vi "Set Averaging.vi"(0 "VISA resource name":refnum<visa-resource-name>, 1 "IF bandwidth (5 : 3000 HZ)":u16(ring)=5 items=["10 HZ", "30 HZ", "100 HZ", "300 HZ", "1000 HZ", "3000 HZ"], 2 "smoothing (F : off)":bool, 5 "average (F : off)":bool, 9 "average factor (16)":u16=16 min=1 max=999, 11 "error in (no error)":errorcluster, 13 "smoothing aperature (1%)":sgl=1.0 min=0.05 max=20 format="%.2f") -> (4 "VISA resource name out":refnum<visa-resource-name>, 15 "error out":errorcluster)   [LabVIEW 2018, in "Agilent 87XX Series.lvlib"]
doc: "This Vi for the HP8753B Network Analyzer is used to set averaging, smoothing, and the IF bandwidth."
uses:
  Agilent 87XX Series.lvlib
panel:
  # "ON\nOFF"
  # "ON\nOFF"
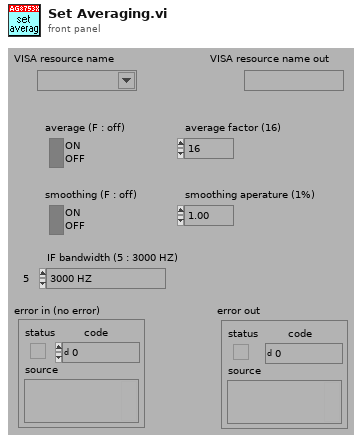
[diagram p1: front panel]
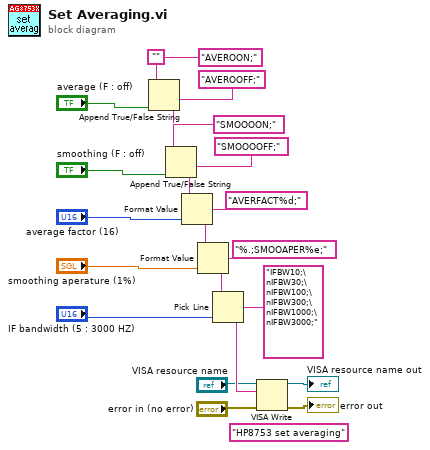
[diagram p0: block diagram]
diagram:
  (unwired) "HP8753 set averaging"
  n1 = Append True/False String(1:"average (F : off)", 2:"AVEROOFF;", 3:"AVEROON;", 4:"") -> (0:w16:string)
  n2 = Append True/False String(1:"smoothing (F : off)", 2:"SMOOOOFF;", 3:"SMOOOON;", 4:w16) -> (0:w14:string)
  n3 = Format Value(string ("")=w14, format string="AVERFACT%d;", value (0)="average factor (16)") -> (output string=w10:string)
  n4 = Format Value(string ("")=w10, format string="%.;SMOOAPER%e;", value (0)="smoothing aperature (1%)") -> (output string=w8:string)
  n5 = Pick Line(string ("")=w8, multi-line string="IFBW10;\nIFBW30;\nIFBW100;\nIFBW300;\nIFBW1000;\nIFBW3000;", line index="IF bandwidth (5 : 3000 HZ)") -> (output string=w5:string)
  n6 = VISA Write(VISA resource name="VISA resource name", write buffer=w5, error in (no error)="error in (no error)") -> (VISA resource name out=→"VISA resource name out":refnum<visa-resource-name>, error out=→"error out":errorcluster)  [unwired: 1 out]
